vi "字符串过滤-数字.vi"(4 "字符串 i":string="1234f将6") -> (0 "全匹配？":bool, 1 "字符串 o":string)   [LabVIEW 2017]
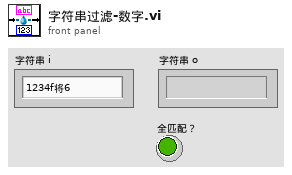
[diagram p1: front panel]
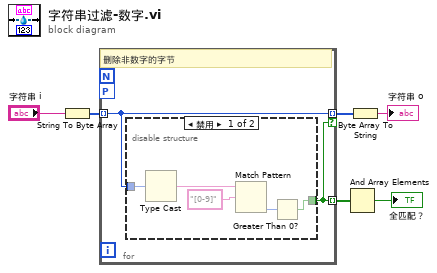
[diagram p0: block diagram]
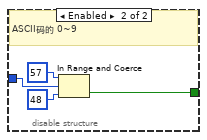
[diagram p2: hidden frame]
diagram:
  n1 = String To Byte Array(string="字符串 i") -> (unsigned byte array=w5:u8[])
  n2 = for {
    tunnel: w5 -> [w8] mode=indexing
    tunnel: [w8] -> w4 mode=indexing if=w7
    workers-P: _ -> [_]
    tunnel: [w7] -> w2 mode=indexing
    # "删除非数字的字节"
    n3 = disable-structure shown="禁用" {
      disable-tunnel: w8 -> [w10 w15]
      disable-tunnel: [w9 w14] -> w7
      frame Disabled {
        n4 = Type Cast(x=w10) -> (*(type *) &x=w13:string)  [unwired: 1 in]
        n5 = Match Pattern(string=w13, regular expression="[0-9]" ("正则表达式")) -> (offset past match=w11:i32)  [unwired: 1 in, 3 out]
        n6 = Greater Than 0?(x=w11) -> (x > 0?=w9:bool)
      }
      frame Enabled {
        # "ASCII码的 0~9"
        n7 = In Range and Coerce(upper limit=u8 57 ("下限"), x=w15, lower limit=u8 48 ("下限")) -> (In Range?=w14:bool)  [unwired: 1 out]
      }
    }
  }
  n8 = And Array Elements(Boolean array=w2) -> (logical AND=→"全匹配？":bool)
  n9 = Byte Array To String(unsigned byte array=w4) -> (string=→"字符串 o":string)
